vi "S2C_UNITHERM_Proc_LocalUpdate.vi"(8 "Error In":errorcluster, 10 "Data":string, 11 "Command":string) -> (0 "Error Out":errorcluster)   [LabVIEW 2015]
uses:
  S2C_UNITHERM_Proc_Globals.vi
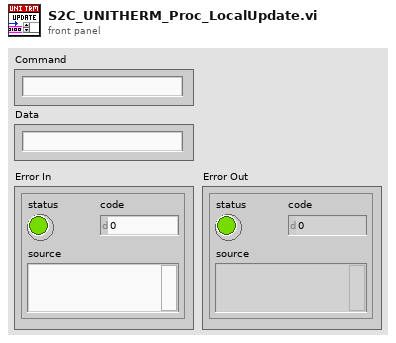
[diagram p1: front panel]
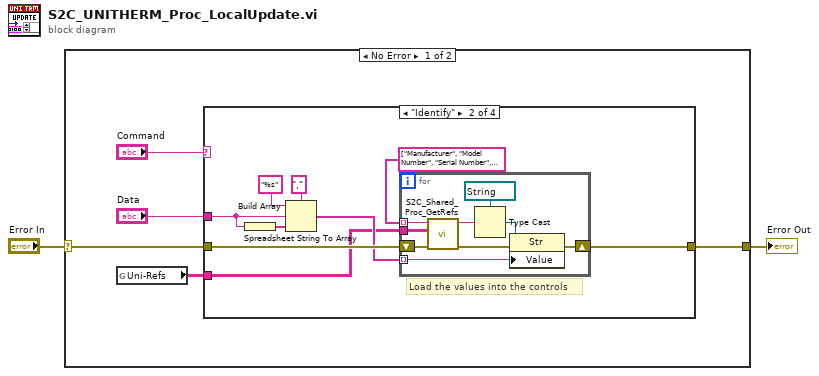
[diagram p0: block diagram]
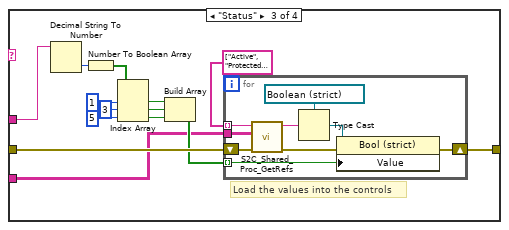
[diagram p3: hidden frame]
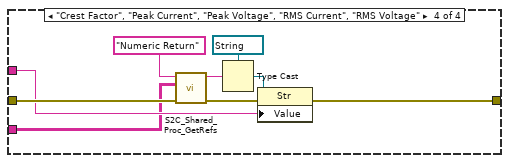
[diagram p4: hidden frame]
diagram:
  n1 = case shown="No Error" "Error In" {
    selector: "Error In" -> [w6 w59]
    tunnel: [w4 w59] -> w1
    frame No Error {
      n2 = global read "S2C_UNITHERM_Proc_Globals.vi" "Uni-Refs"() -> (w3:string[][])
      n3 = case shown="\"Identify\"" "Command" {
        tunnel: w6 -> [w8 w13 w40 w54]
        tunnel: "Data" -> [_ w14 w36 w52]
        tunnel: [w8 w10 w38 w53] -> w4
        tunnel: w3 -> [_ w9 w27 w50]
        frame "Other", Default {
        }
        frame "Identify" {
          # "Load the values into the controls"
          n4 = Build Array(w14) -> (w15:string[])
          n5 = Spreadsheet String To Array(delimiter (Tab)=",", format string="%s", spreadsheet string=w14, array type (2D Dbl)=w15) -> (array=w12:string[])
          n6 = for {
            tunnel: w12 -> [w20] mode=indexing
            tunnel: string[] ["Manufacturer", "Model Number", "Serial Number", "Firmware Version"] -> [w21] mode=indexing
            shift-right: [w19] -> w10
            shift-left: w13 -> [w22]
            tunnel: w9 -> [w18]
            n7 = call "S2C_Shared_Proc_GetRefs.vi"("Error In"=w22, "Refs"=w18, "Label"=w21) -> ("Error Out"=w25:errorcluster, "Reference"=w23:string)  [unwired: 7 in]
            n8 = Type Cast(type=refnum<vi> refnum ("Enum"), x=w23) -> (*(type *) &x=w24:refnum<vi>)
            n9 = property class="Str"(reference=w24, error in=w25, "Value"=w20) -> (error out=w19:errorcluster)  [unwired: 1 out]
          }
        }
        frame "Status" {
          # "Load the values into the controls"
          n10 = Decimal String To Number(string=w36) -> (number=w37:i32)  [unwired: 2 in, 1 out]
          n11 = Number To Boolean Array(number=w37) -> (Boolean array=w29:bool[])
          n12 = Index Array(array=w29, index #1=1 ("index"), index #2=3 ("index"), index #3=5 ("index")) -> (element #1=w30:bool, element #2=w31:bool, element #3=w32:bool)
          n13 = Build Array(w30, w31, w32) -> (w28:bool[])
          n14 = for {
            tunnel: w28 -> [w44] mode=indexing
            tunnel: string[] ["Active", "Protected", "Disconnected"] -> [w45] mode=indexing
            shift-right: [w43] -> w38
            shift-left: w40 -> [w46]
            tunnel: w27 -> [w41]
            n15 = call "S2C_Shared_Proc_GetRefs.vi"("Error In"=w46, "Refs"=w41, "Label"=w45) -> ("Error Out"=w49:errorcluster, "Reference"=w47:string)  [unwired: 7 in]
            n16 = Type Cast(type=refnum<vi> refnum ("Boolean"), x=w47) -> (*(type *) &x=w48:refnum<vi>)
            n17 = property class="Bool (strict)"(reference=w48, error in=w49, "Value"=w44) -> (error out=w43:errorcluster)  [unwired: 1 out]
          }
        }
        frame "Crest Factor", "Peak Current", "Peak Voltage", "RMS Current", "RMS Voltage" {
          n18 = call "S2C_Shared_Proc_GetRefs.vi"("Error In"=w54, "Refs"=w50, "Label"="Numeric Return") -> ("Error Out"=w57:errorcluster, "Reference"=w55:string)  [unwired: 7 in]
          n19 = Type Cast(type=refnum<vi> refnum ("Enum"), x=w55) -> (*(type *) &x=w56:refnum<vi>)
          n20 = property class="Str"(reference=w56, error in=w57, "Value"=w52) -> (error out=w53:errorcluster)  [unwired: 1 out]
        }
      }
    }
    frame Error {
    }
  }
  "Error Out" <- w1
